vi "Send CCD Initialization.vi"(8 "error in (no error)":errorcluster, 11 "Stream in":refnum<class "Stream.lvclass">) -> (0 "error out":errorcluster, 3 "Stream out":refnum<class "Stream.lvclass">)   [LabVIEW 2018, in "Stream.lvclass"]
uses:
  Stream.lvclass
  Stream.lvclass/Stream.ctl
  Interface/Interface.lvclass/Interface.ctl
  Interface/Interface.lvclass
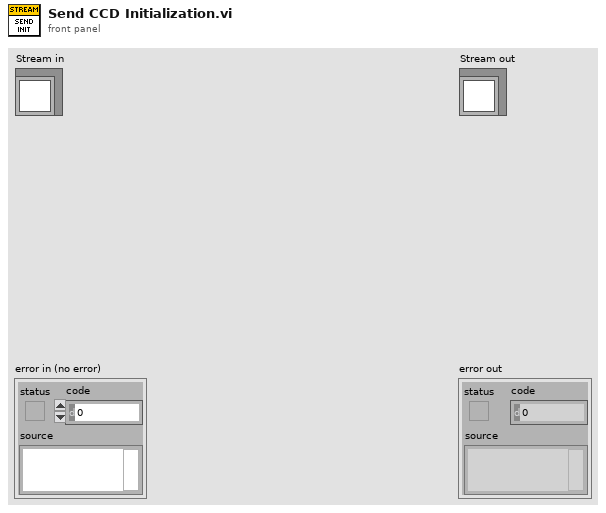
[diagram p1: front panel]
types:
  T1 = cluster{"Initialization":bool, "Serial Number":u16}
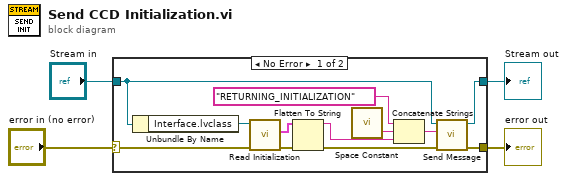
[diagram p0: block diagram]
diagram:
  n1 = case shown="No Error" "error in (no error)" {
    selector: "error in (no error)" -> [w14 w18]
    tunnel: [w12 w18] -> w3
    tunnel: [w6 w17] -> w1
    tunnel: "Stream in" -> [w5 w17]
    frame No Error {
      n2 = Unbundle By Name(w5) -> ("Interface.lvclass"=w16:refnum<class "Interface.lvclass">)
      n3 = call "Read Initialization.vi"("error in (no error)"=w14, "Interface in"=w16) -> ("error out"=w13:errorcluster, "Initialization"=w15:T1)  [unwired: 7 in, 1 out]
      n4 = Flatten To String(anything=w15, error in (no error)=w13) -> (data string=w8:string, error out=w11:errorcluster)  [unwired: 2 in, 1 out]
      n5 = call <vilib>:"Space Constant.vi"() -> ("String"=w9:string)
      n6 = Concatenate Strings("RETURNING_INITIALIZATION" ("string"), w9, w8) -> (w7:string)
      n7 = call "Send Message.vi"("error in (no error)"=w11, "Message"=w7, "Stream in"=w5) -> ("error out"=w12:errorcluster, "Stream out"=w6:refnum<class "Stream.lvclass">)  [unwired: 7 in]
    }
    frame Error {
    }
  }
  "error out" <- w3
  "Stream out" <- w1
